vi "CSM Execute - Remove all CSM Bookmarks.vi"(6 "Mouse Position":T1, 8 "User VI Ref":refnum<vi>, 9 "Menu Item Tag Suffix":string, 10 "Remaining Items":refnum<vi>[](array[refnum]), 11 "Affected Items":T2) -> (0 "Fail transaction?":bool)   [LabVIEW 2017]
doc: "This VI is part of a plug-in for modifying the LabVIEW shortcut menus. This is the execute VI which is called when the shortcut menu is chosen by the user. It performs the action of the selected menu item."
uses:
  CSM Execute - Shortcut Menu Plug-In.ctl
  <vilib>/Utility/miscctls.llb/LVPositionTypeDef.ctl
  _csmHelper/API/Destroy.vi
  _csmHelper/usecase/Remove All CSM Bookmarks.vi
  _csmHelper/API/Open Block Diagram.vi
  _csmHelper/API/Create From VI Reference.vi
  _csmHelper/CSM-Helper.lvclass
panel:
  # "All controls on this panel except \"Affected Items\" have been locked to prevent accidental edits. Changing the control names or types, other than the elements of the \"Affected Items\" cluster will make the VI unusable as a menu plugin.\n\nSee Context Help for each control for details about its use."
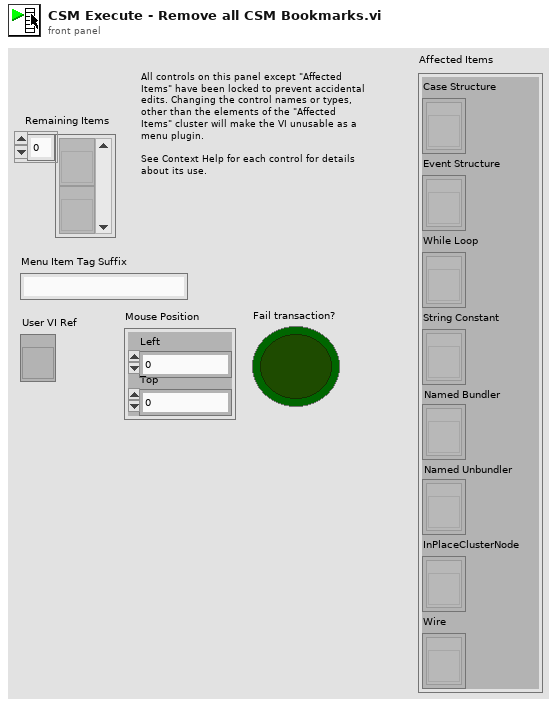
[diagram p1: front panel]
types:
  T1 = typedef "LVPositionTypeDef.ctl" = cluster{"Left":i32, "Top":i32}
  T2 = typedef "CSM Execute - Shortcut Menu Plug-In.ctl" = cluster{"Case Structure":refnum<vi>[], "Event Structure":refnum<vi>[], "While Loop":refnum<vi>[], "String Constant":refnum<vi>[], "Named Bundler":refnum<vi>[], "Named Unbundler":refnum<vi>[], "InPlaceClusterNode":refnum<vi>[], "Wire":refnum<vi>[]}
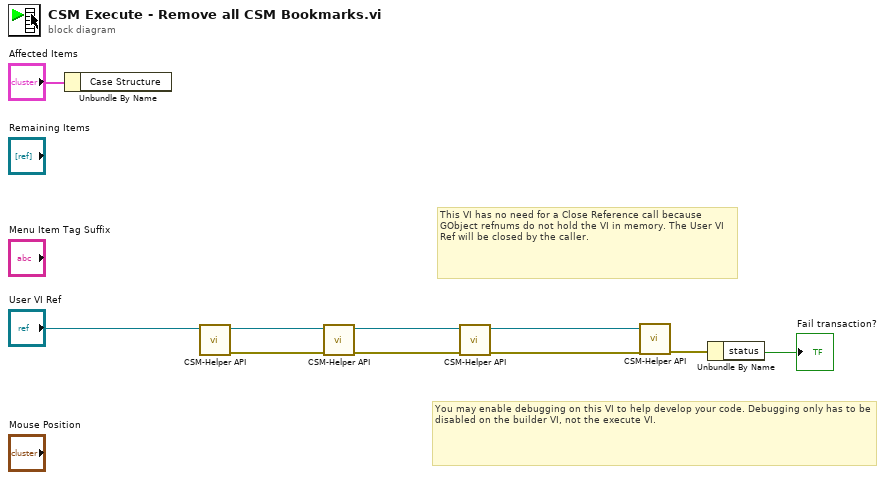
[diagram p0: block diagram]
diagram:
  # "You may enable debugging on this VI to help develop your code. Debugging only has to be disabled on the builder VI, not the execute VI."
  # "This VI has no need for a Close Reference call because GObject refnums do not hold the VI in memory. The User VI Ref will be closed by the caller."
  n1 = Unbundle By Name("Affected Items") -> ()  [unwired: 1 out]
  n2 = call-poly "CSM-Helper API.vi"("VI"="User VI Ref") -> ("error out"=w8:errorcluster, "CSM-Helper.lvclass"=w7:refnum<class "CSM-Helper.lvclass">)  [unwired: 9 in]
  n3 = call-poly "CSM-Helper API.vi"("error in (no error)"=w8, "CSM-Helper in"=w7) -> ("error out"=w6:errorcluster, "CSM-Helper out"=w5:refnum<class "CSM-Helper.lvclass">)  [unwired: 8 in]
  n4 = call-poly "CSM-Helper API.vi"("error in (no error)"=w6, "CSM-Helper in"=w5) -> ("error out"=w4:errorcluster, "CSM-Helper out"=w3:refnum<class "CSM-Helper.lvclass">)  [unwired: 8 in]
  n5 = call-poly "CSM-Helper API.vi"("error in (no error)"=w4, "CSM-Helper in"=w3) -> ("error out"=w1:errorcluster)  [unwired: 8 in, 1 out]
  n6 = Unbundle By Name(w1) -> ("status"=→"Fail transaction?":bool)
